vi "Prepare Paths For Expiration Check.vi"(0 "Path Groups in":refnum<class "Path Group.lvclass">[](array[class]), 5 "TSM Context":T1, 11 "error in":errorcluster) -> (4 "Path Groups out":refnum<class "Path Group.lvclass">[](array[class]), 15 "error out":errorcluster)   [LabVIEW 2023, in "RFFixtureCharact.Public.lvlib"]
uses:
  RFFixtureCharact.Public.lvlib
  <vilib>/NI_TestStand_SemiconductorModule/NI_TestStand_Semiconductor_Module.lvlibp/PinMap/General/SemiconductorModuleContext.ctl
  Common/Base Classes/Path Group/Path Group.lvclass
  Common/RFCalAndFixtureCharact.Common.lvlib
  <vilib>/NI_TestStand_SemiconductorModule/NI_TestStand_Semiconductor_Module.lvlibp
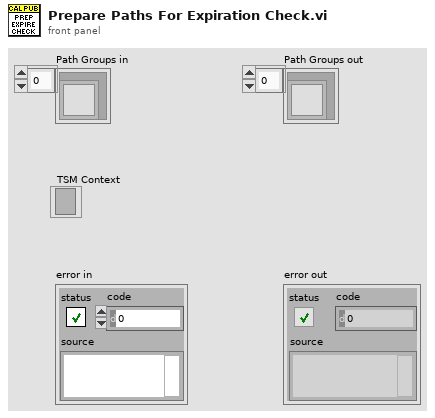
[diagram p1: front panel]
types:
  T1 = typedef "NI_TestStand_Semiconductor_Module.lvlibp/SemiconductorModuleContext.ctl" = refnum<k7>
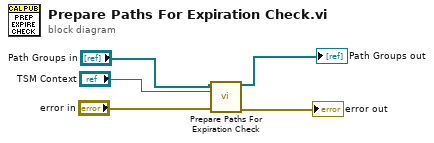
[diagram p0: block diagram]
diagram:
  n1 = call "Prepare Paths For Expiration Check.vi"("Path Groups in"="Path Groups in", "TSM Context"="TSM Context", "error in (no error)"="error in") -> ("Path Groups out"=→"Path Groups out":refnum<class "Path Group.lvclass">[], "error out"=→"error out":errorcluster)  [unwired: 11 in]
